vi "Level Units To Text (G3).vi"(8 "error in (no error)":errorcluster, 11 "Level":T1) -> (0 "error out":errorcluster, 3 "String":string)   [LabVIEW 2020]
uses:
  Level Data.ctl
  Level Units (G3).ctl
  Level (G3).xctl
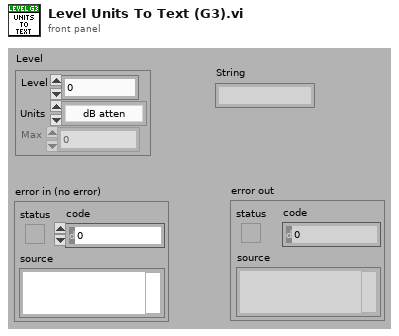
[diagram p1: front panel]
types:
  T1 = typedef "Level (G3).xctl/Level Data.ctl" = cluster{"Level":dbl, "Units":T2, "Max":dbl, "Data":cluster{"Multiplier":dbl, "Cal File":path, "Cal":cluster{"Freq (Hz)":dbl[], "Mag (dB SPL)":dbl[], "Phase (deg)":dbl[]}, "audiogram":path}}
  T2 = typedef "Level (G3).xctl/Level Units (G3).ctl" = enum16{"dB atten", "dB SPL", "dB re 1 Vrms", "dB V/Hz½", "mW", "dB HL", "Volts", "dB mW"}
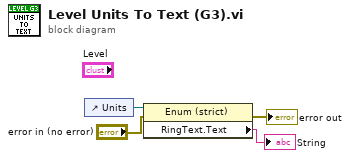
[diagram p0: block diagram]
diagram:
  n1 = control-ref of="Units"() -> (w3:refnum<vi>)
  n2 = property class="Enum (strict)"(reference=w3, error in="error in (no error)") -> (error out=→"error out":errorcluster, "RingText.Text"=→"String":string)  [unwired: 1 out]
